vi "LowBarAuto.vi"(8 "error in (no error)":errorcluster) -> (0 "Terminate":bool)   [LabVIEW 2015]
uses:
  Utilities/VisionGlobals.vi
  Utilities/ShiftGlobals.vi
  Utilities/GlobalVisionVars.vi
  Utilities/MotorPositionGlobals.vi
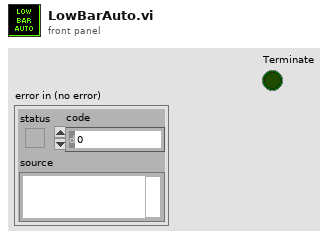
[diagram p1: front panel]
types:
  T1 = typedef "WPI_MotorControlDeviceRef.ctl" = cluster{"DeviceStatus":errorcluster, "Type":T2, "PWM":cluster{"PWM Channel":T3, "DeadBand":T4}, "CAN":cluster{"Device Number":u8, "Control Mode":T5, "Semaphore":T6, "Max Vout":dbl, "TalonSRX Control Mode":T7}, "Invert":bool}
  T2 = typedef "WPI_MotorControlType.ctl" = enum16{"PWM", "CAN", "CANTalonSRX"}
  T3 = typedef "FPGA_DIOPWMChannel.ctl" = enum8{"PWM 0", "PWM 1", "PWM 2", "PWM 3", "PWM 4", "PWM 5", "PWM 6", "PWM 7", "PWM 8", "PWM 9", "PWM MXP 0", "PWM MXP 1", "PWM MXP 2", "PWM MXP 3", "PWM MXP 4", "PWM MXP 5", "PWM MXP 6", "PWM MXP 7", "PWM MXP 8", "PWM MXP 9", "Invalid"}
  T4 = typedef "WPI_PWMDeadband.ctl" = cluster{"Name":string, "maxPositivePwm":i32, "minPositivePwm":i32, "centerPwm":i32, "maxNegativePwm":i32, "minNegativePwm":i32, "angularRange":u16}
  T5 = typedef "WPI_CANJaguar_ControlMode.ctl" = enum8{"Percent VBus", "Current", "Speed", "Position", "Voltage"}
  T6 = typedef "Semaphore RefNum" = refnum<k1>
  T7 = typedef "WPI_CANTalonSRX_APIControlMode.ctl" = enum8{"Percent VBus", "Speed", "Position", "Slave", "Unchanged / Invalid", "Voltage Compensation", "Current", "Motion Profile"}
  T8 = typedef "WPI_CANTalonSRX_GlobalStatus.ctl" = cluster{"Applied Throttle":dbl, "Module Enabled":bool, "CAN Error":errorcluster, "Closed Loop Error":dbl, "Forward Limit Switch Closed":bool, "Reverse Limit Switch Closed":bool, "Sensor Position":dbl, "Sensor Velocity":dbl, "Current":dbl, "Sticky Fault - Over Temp":bool, "Sticky Fault - Under Voltage":bool, "Sticky Fault - Forward Limit":bool, "Sticky Fault - Reverse Limit":bool, "Sticky Fault - Forward Soft Limit":bool, "Sticky Fault - Reverse Soft Limit":bool, "Brake is Enabled":bool, "Encoder Position":dbl, "Encoder Velocity":dbl, "Encoder Index Count":dbl, "Encoder A Pin State":bool, "Encoder B Pin State":bool, "Encoder Index Pin State":bool, "Analog In":dbl, "Analog In Velocity":dbl, "Temperature (C)":dbl, "Battery Voltage":dbl, "Control 5 Is Supported":bool, "Current Profile Slot Select":dbl, "Pos Div 8":bool, "Vel Div 4":bool, "Pulse Width Position":i32, "Pulse Width Velocity":i32, "Pulse Width Rise To Rise (us)":i32, "Pulse Width Rise To Fall (us)":i32, "Mot Prof Active Is Under Run":bool, "Mot Prof Active Has Under Run":bool, "Mot Prof Active Is Last":bool, "Mot Prof Active Velocity Only":bool, "Mot Prof Active Is Valid":bool, "Mot Prof Buffer Is Full":bool, "Mot Prof Active Profile Slot Select":i32, "Mot Prof NextID":i32, "Mot Prof Count":i32, "Mot Prof Active Velocity":dbl, "Mot Prof Active Position":dbl, "Mot Prof Output Enable":i32}
  T9 = typedef "WPI_DigitalOutputDevRef.ctl" = cluster{"DIO Channel":T10, "DevStatus":errorcluster}
  T10 = typedef "FPGA_DIOChannel.ctl" = enum8{"DIO 0", "DIO 1", "DIO 2", "DIO 3", "DIO 4", "DIO 5", "DIO 6", "DIO 7", "DIO 8", "DIO 9", "DIO MXP 0", "DIO MXP 1", "DIO MXP 2", "DIO MXP 3", "DIO MXP 4", "DIO MXP 5", "DIO MXP 6", "DIO MXP 7", "DIO MXP 8", "DIO MXP 9", "DIO MXP 10", "DIO MXP 11", "DIO MXP 12", "DIO MXP 13", "DIO MXP 14", "DIO MXP 15", "Invalid"}
  T11 = typedef "WPI_GyroDevRef.ctl" = cluster{"DevStatus":errorcluster, "Analog Channel":T12, "Offset":dbl, "Gain (VoltsPerDegree/Second)":dbl, "Gyro Type":enum16{"Analog", "XRS450"}, "Handle":i32, "SPI Bus":T13, "Device Found":bool, "Sample Rate":dbl, "Calibrate On Open":bool}
  T12 = typedef "FPGA_AIChannel.ctl" = enum8{"AI 0", "AI 1", "AI 2", "AI 3", "AI MXP 0", "AI MXP 1", "AI MXP 2", "AI MXP 3", "Invalid"}
  T13 = typedef "spi_bus.ctl" = enum16{"SPI On-Board, CS0", "SPI On-Board, CS1", "SPI On-Board, CS2", "SPI On-Board, CS3", "SPI MXP", "Invalid"}
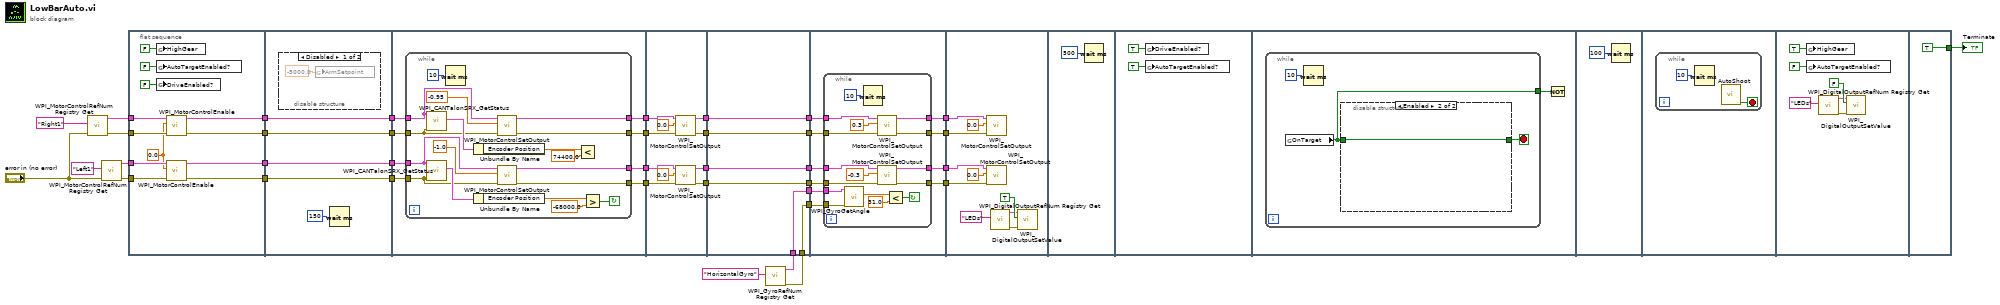
[diagram p0: block diagram]
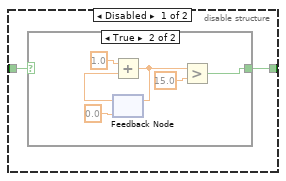
[diagram p3: hidden frame]
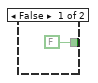
[diagram p4: hidden frame]
diagram:
  n1 = call <vilib>:"WPI_MotorControlRefNum Registry Get.vi"("error in (no error)"="error in (no error)", "refnum name"="Right1") -> ("error out"=w31:errorcluster, "MotorControlDevRef"=w32:T1)  [unwired: 8 in]
  n2 = call <vilib>:"WPI_MotorControlRefNum Registry Get.vi"("error in (no error)"="error in (no error)", "refnum name"="Left1") -> ("error out"=w33:errorcluster, "MotorControlDevRef"=w34:T1)  [unwired: 8 in]
  n3 = flat-sequence {
    tunnel: w31 -> [w44]
    tunnel: w32 -> [w46]
    tunnel: w33 -> [w41]
    tunnel: w34 -> [w42]
    tunnel: [w40] -> w26
    tunnel: [w39] -> w24
    tunnel: [w45] -> w22
    tunnel: [w43] -> w20
    tunnel: w26 -> [w54]
    tunnel: [w54] -> w25
    tunnel: w24 -> [w53]
    tunnel: [w53] -> w23
    tunnel: w22 -> [w52]
    tunnel: [w52] -> w21
    tunnel: w20 -> [w51]
    tunnel: [w51] -> w19
    tunnel: w19 -> [w60]
    tunnel: w21 -> [w61]
    tunnel: w23 -> [w62]
    tunnel: w25 -> [w63]
    tunnel: [w59] -> w18
    tunnel: [w58] -> w17
    tunnel: [w57] -> w16
    tunnel: [w56] -> w15
    tunnel: [w89] -> w13
    tunnel: [w88] -> w11
    tunnel: [w87] -> w9
    tunnel: [w86] -> w7
    tunnel: w18 -> [w85]
    tunnel: w17 -> [w84]
    tunnel: w16 -> [w83]
    tunnel: w15 -> [w82]
    tunnel: w13 -> [w97]
    tunnel: [w97] -> w12
    tunnel: w11 -> [w96]
    tunnel: [w96] -> w10
    tunnel: w9 -> [w95]
    tunnel: [w95] -> w8
    tunnel: w7 -> [w94]
    tunnel: [w94] -> w6
    tunnel: w5 -> [w93]
    tunnel: [w93] -> w4
    tunnel: w3 -> [w92]
    tunnel: [w92] -> w2
    tunnel: w12 -> [w107]
    tunnel: w10 -> [w106]
    tunnel: w8 -> [w105]
    tunnel: w6 -> [w104]
    tunnel: [w103] -> w30
    tunnel: [w102] -> w29
    tunnel: [w101] -> w28
    tunnel: [w100] -> w27
    tunnel: w4 -> [w99]
    tunnel: w2 -> [w98]
    tunnel: w30 -> [w131]
    tunnel: w29 -> [w130]
    tunnel: w28 -> [w129]
    tunnel: w27 -> [w128]
    tunnel: [TRUE] -> w1
    frame #0 {
      w38 = 0.0 ("Encoder Initial Position")
      n4 = global write "ShiftGlobals.vi" "HighGear"(FALSE ("HighGear")) -> ()
      n5 = global write "VisionGlobals.vi" "AutoTargetEnabled?"(FALSE ("AutoTargetEnabled?")) -> ()
      n6 = global write "VisionGlobals.vi" "DriveEnabled?"(FALSE ("DriveEnabled?")) -> ()
      n7 = call <vilib>:"WPI_MotorControlEnable.vi"("error in (no error)"=w44, "Encoder Initial Position"=w38, "CAN MotorDevRef"=w46) -> ("error out"=w43:errorcluster, "CAN MotorDevRef"=w45:T1)  [unwired: 7 in]
      n8 = call <vilib>:"WPI_MotorControlEnable.vi"("error in (no error)"=w41, "Encoder Initial Position"=w38, "CAN MotorDevRef"=w42) -> ("error out"=w39:errorcluster, "CAN MotorDevRef"=w40:T1)  [unwired: 7 in]
    }
    frame #1 {
      n9 = disable-structure shown="Disabled" {
        frame Disabled {
          n10 = global write "MotorPositionGlobals.vi" "ArmSetpoint"(-5000.0 ("ArmSetpoint")) -> ()
        }
        frame Enabled {
        }
      }
      n11 = Wait (ms)(milliseconds to wait=u32 150) -> ()  [unwired: 1 out]
    }
    frame #2 {
      n12 = while {
        tunnel: w63 -> [w66]
        tunnel: w62 -> [w65]
        tunnel: w61 -> [w68]
        tunnel: w60 -> [w67]
        tunnel: [w74] -> w59
        tunnel: [w73] -> w58
        tunnel: [w72] -> w57
        tunnel: [w71] -> w56
        stop <- w64 continue-if-true
        n13 = call <vilib>:"WPI_CANTalonSRX_GetStatus.vi"("error in (no error)"=w67, "CAN Talon SRX Ref"=w68) -> ("Talon SRX Status"=w79:T8)  [unwired: 7 in, 2 out]
        n14 = call <vilib>:"WPI_CANTalonSRX_GetStatus.vi"("error in (no error)"=w65, "CAN Talon SRX Ref"=w66) -> ("Talon SRX Status"=w78:T8)  [unwired: 7 in, 2 out]
        n15 = Wait (ms)(milliseconds to wait=u32 10) -> ()  [unwired: 1 out]
        n16 = Unbundle By Name(w79) -> ("Encoder Position"=w77:dbl)
        n17 = Unbundle By Name(w78) -> ("Encoder Position"=w76:dbl)
        n18 = call <vilib>:"WPI_MotorControlSetOutput.vi"("error in (no error)"=w67, "Output"=-0.95, "MotorControlDevRef"=w68) -> ("error out"=w71:errorcluster, "MotorControlDevRef"=w72:T1)  [unwired: 6 in, 1 out]
        n19 = call <vilib>:"WPI_MotorControlSetOutput.vi"("error in (no error)"=w65, "Output"=-1.0, "MotorControlDevRef"=w66) -> ("error out"=w73:errorcluster, "MotorControlDevRef"=w74:T1)  [unwired: 6 in, 1 out]
        n20 = Less?(x=w77, y=74400.0) -> ()  [unwired: 1 out]
        n21 = Greater?(x=w76, y=-68000.0) -> (0:w64:bool)
      }
    }
    frame #3 {
      n22 = call <vilib>:"WPI_MotorControlSetOutput.vi"("error in (no error)"=w82, "Output"=0.0, "MotorControlDevRef"=w83) -> ("error out"=w86:errorcluster, "MotorControlDevRef"=w87:T1)  [unwired: 6 in, 1 out]
      n23 = call <vilib>:"WPI_MotorControlSetOutput.vi"("error in (no error)"=w84, "Output"=0.0, "MotorControlDevRef"=w85) -> ("error out"=w88:errorcluster, "MotorControlDevRef"=w89:T1)  [unwired: 6 in, 1 out]
    }
    frame #4 {
    }
    frame #5 {
      n24 = while {
        tunnel: w107 -> [w121]
        tunnel: w106 -> [w120]
        tunnel: w105 -> [w119]
        tunnel: w104 -> [w118]
        tunnel: [w117] -> w103
        tunnel: [w116] -> w102
        tunnel: [w115] -> w101
        tunnel: [w114] -> w100
        tunnel: w99 -> [w113]
        tunnel: w98 -> [w112]
        stop <- w109 continue-if-true
        n25 = call <vilib>:"WPI_GyroGetAngle.vi"("error in"=w112, "GyroDevRef"=w113) -> ("Angle"=w111:dbl)  [unwired: 5 in, 4 out]
        n26 = Wait (ms)(milliseconds to wait=u32 10) -> ()  [unwired: 1 out]
        n27 = call <vilib>:"WPI_MotorControlSetOutput.vi"("error in (no error)"=w118, "Output"=0.3, "MotorControlDevRef"=w119) -> ("error out"=w114:errorcluster, "MotorControlDevRef"=w115:T1)  [unwired: 6 in, 1 out]
        n28 = call <vilib>:"WPI_MotorControlSetOutput.vi"("error in (no error)"=w120, "Output"=-0.3, "MotorControlDevRef"=w121) -> ("error out"=w116:errorcluster, "MotorControlDevRef"=w117:T1)  [unwired: 6 in, 1 out]
        n29 = Less?(x=w111, y=31.0) -> (x < y?=w109:bool)
      }
    }
    frame #6 {
      n30 = call <vilib>:"WPI_MotorControlSetOutput.vi"("error in (no error)"=w128, "Output"=0.0, "MotorControlDevRef"=w129) -> ()  [unwired: 6 in, 3 out]
      n31 = call <vilib>:"WPI_MotorControlSetOutput.vi"("error in (no error)"=w130, "Output"=0.0, "MotorControlDevRef"=w131) -> ()  [unwired: 6 in, 3 out]
      n32 = call <vilib>:"WPI_DigitalOutputRefNum Registry Get.vi"("refnum name"="LEDs") -> ("error out"=w126:errorcluster, "DigitalOutputDevRef"=w125:T9)  [unwired: 9 in]
      n33 = call <vilib>:"WPI_DigitalOutputSetValue.vi"("error in (no error)"=w126, "Value"=TRUE, "DigitalOutputDevRef"=w125) -> ()  [unwired: 7 in, 2 out]
    }
    frame #7 {
      n34 = Wait (ms)(milliseconds to wait=u32 500) -> ()  [unwired: 1 out]
    }
    frame #8 {
      n35 = global write "VisionGlobals.vi" "DriveEnabled?"(TRUE ("DriveEnabled?")) -> ()
      n36 = global write "VisionGlobals.vi" "AutoTargetEnabled?"(TRUE ("AutoTargetEnabled?")) -> ()
    }
    frame #9 {
      n37 = while {
        tunnel: [w138] -> w137
        stop <- w139 stop-if-true
        n38 = global read "GlobalVisionVars.vi" "OnTarget"() -> (w138:bool)
        n39 = Wait (ms)(milliseconds to wait=u32 10) -> ()  [unwired: 1 out]
        n40 = disable-structure shown="Enabled" {
          disable-tunnel: [w142 w150] -> w139
          disable-tunnel: w138 -> [w141 w150]
          frame Disabled {
            n41 = case shown="True" w141 {
              tunnel: [FALSE w144] -> w142
              frame False {
              }
              frame True {
                n42 = feedback #1(0.0) -> (w148:dbl)
                n43 = Add(x=1.0, y=w148) -> (x+y=w146:dbl)
                n44 = feedback-in #1(w146) -> ()
                n45 = Greater?(x=w146, y=15.0) -> (0:w144:bool)
              }
            }
          }
          frame Enabled {
          }
        }
      }
      n46 = Not(x=w137) -> ()  [unwired: 1 out]
    }
    frame #10 {
      n47 = Wait (ms)(milliseconds to wait=u32 100) -> ()  [unwired: 1 out]
    }
    frame #11 {
      n48 = while {
        stop <- w152 stop-if-true
        n49 = Wait (ms)(milliseconds to wait=u32 10) -> ()  [unwired: 1 out]
        n50 = call "AutoShoot.vi"() -> ("Terminate"=w152:bool)  [unwired: 11 in]
      }
    }
    frame #12 {
      n51 = global write "ShiftGlobals.vi" "HighGear"(TRUE ("HighGear")) -> ()
      n52 = global write "VisionGlobals.vi" "AutoTargetEnabled?"(FALSE ("AutoTargetEnabled?")) -> ()
      n53 = call <vilib>:"WPI_DigitalOutputRefNum Registry Get.vi"("refnum name"="LEDs") -> ("error out"=w157:errorcluster, "DigitalOutputDevRef"=w156:T9)  [unwired: 9 in]
      n54 = call <vilib>:"WPI_DigitalOutputSetValue.vi"("error in (no error)"=w157, "Value"=FALSE, "DigitalOutputDevRef"=w156) -> ()  [unwired: 7 in, 2 out]
    }
    frame #13 {
    }
  }
  n55 = call <vilib>:"WPI_GyroRefNum Registry Get.vi"("refnum name"="HorizontalGyro") -> ("error out"=w3:errorcluster, "GyroDevRef"=w5:T11)  [unwired: 9 in]
  "Terminate" <- w1
